vi "Control - X-tau.vi"(8 "Control Inputs":T1 {"CA50 Control Output [CAD]" format="%.2f"; "Exhaust Manifold Temp [C]" format="%#_6f"; "UEGO2Lambda" format="%.2f"; "Intake Manifold Temp (MAT) [C]" format="%#_6f"; "UEGO1Lambda" format="%.2f"}, 11 "Fuel Mass [mg/cyc]":sgl) -> (3 "Fuel Mass [mg/cyc]":sgl)   [LabVIEW 2015, in "ECS-RT.lvlib"]
uses:
  ECS-RT.lvlib
  Typedefs/Control Inputs/Control Inputs.ctl
  Typedefs/EPT/Engine Status.ctl
  Typedefs/MISC/Load Control Mode.ctl
  ECS-Shared.lvlib
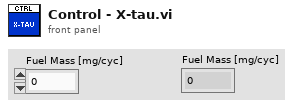
[diagram p1: front panel]
types:
  T1 = typedef "ECS-Shared.lvlib/Control Inputs.ctl" = cluster{"Engine Speed [RPM]":sgl, "Engine Status":T2, "Load Control \nMode":T3, "dt(s)":sgl, "Number of Cylinders":u8, "Engine Displacement [cc]":sgl, "StoichAFR":sgl, "Q.LHV Fuel [kJ/kg]":sgl, "BattV PSU [V]":sgl, "12V PSU [V]":sgl, "5V PSU [V]":sgl, "Pedal Position [%]":sgl, "Oil Pressure [kPa]":sgl, "Oil Temp [C]":sgl, "Oil Level [%]":sgl, "Engine Coolant Temp (ECT) [C]":sgl, "Engine Coolant Pressure [kPa]":sgl, "Rail Pressure [bar]":sgl, "Fuel Pressure [kPa]":sgl, "Fuel Temp [C]":sgl, "Vacuum Pressure [kPa]":sgl, "Throttle Position [%]":sgl, "Cam1 Advance [CAD]":sgl, "Cam2 Advance [CAD]":sgl, "CA50 Control Output [CAD]":sgl[], "CA50 Control Output Valid":bool[], "Intake Air Temp (IAT) [C]":sgl, "Barometric Air Pressure [kPa]":sgl, "Intake Air Rel. Humidity [%]":sgl, "Mass Air Flow (MAF) [kg/hr]":sgl, "Turbo Inlet Air Pressure [kPa]":sgl, "Turbo Inlet Air Temp [C]":sgl, "Turbo Outlet Air Pressure [kPa]":sgl, "Turbo Outlet Air Temp [C]":sgl, "CAC Outlet Pressure [kPa]":sgl, "CAC Outlet Temp [C]":sgl, "Intake Manifold Pressure (MAP) [kPa]":sgl, "Intake Manifold Temp (MAT) [C]":sgl, "Exhaust Manifold Pressure [kPa]":sgl, "Exhaust Manifold Temp [C]":sgl, "HighP EGR Cooler Outlet Pressure [kPa]":sgl, "HighP EGR Cooler Outlet Temp [C]":sgl, "HighP EGR Differential Pressure [kPa]":sgl, "HighP EGR Valve Position [%]":sgl, "Turbo Outlet Exhaust Pressure [kPa]":sgl, "Turbo Outlet Exhaust Temp [C]":sgl, "VGT Position 1 [%]":sgl, "VGT Position 2 [%]":sgl, "Turbo Speed 1 [RPM]":sgl, "Turbo Speed 2 [RPM]":sgl, "LowP EGR Differential Pressure [kPa]":sgl, "LowP EGR Valve Position [%]":sgl, "UEGO1Lambda":sgl, "UEGO1_Hot":bool, "UEGO2Lambda":sgl, "UEGO2_Hot":bool}
  T2 = typedef "ECS-Shared.lvlib/Engine Status.ctl" = enum16{"STALLED", "CRANKING", "RUNNING", "ACCEL", "DECEL", "SAFE", "OFF"}
  T3 = typedef "ECS-Shared.lvlib/Load Control Mode.ctl" = enum16{"No Governor", "Low-Idle Governor", "High-Idle Governor"}
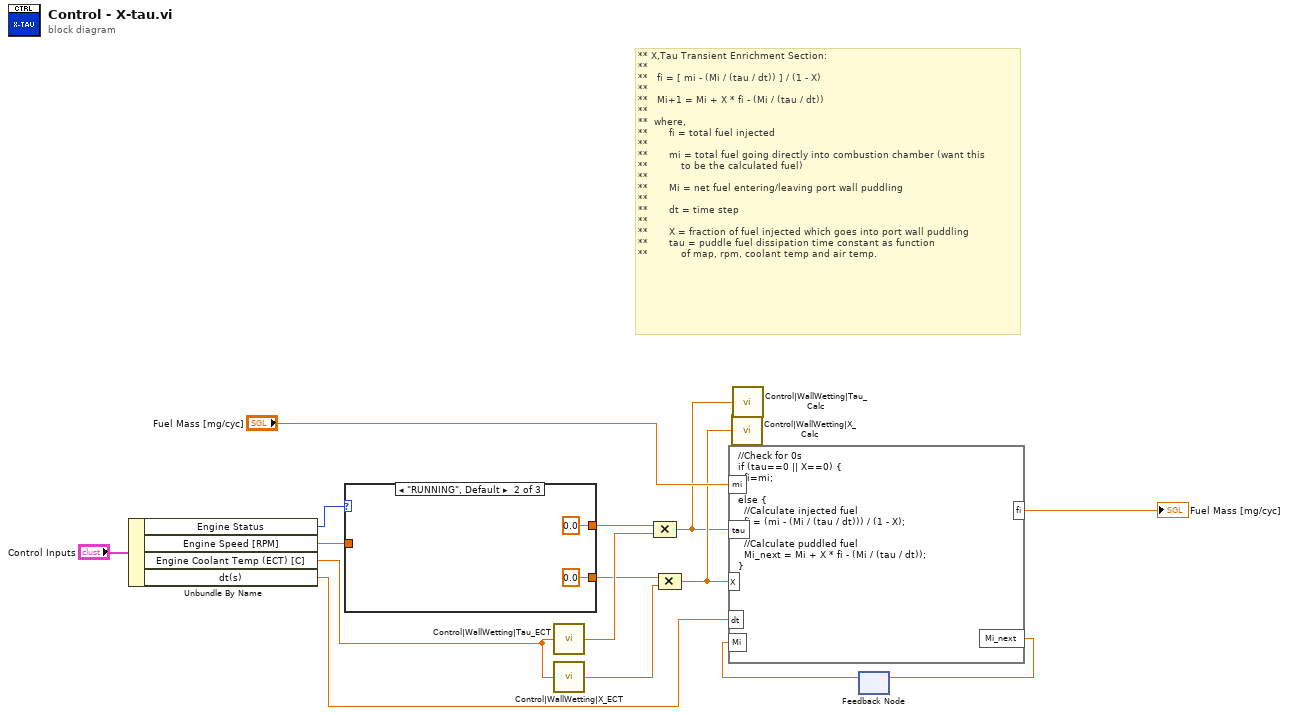
[diagram p0: block diagram]
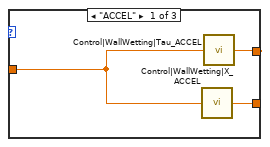
[diagram p2: hidden frame]
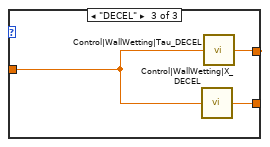
[diagram p3: hidden frame]
diagram:
  # "** X,Tau Transient Enrichment Section:\n**   \n**   fi = [ mi - (Mi / (tau / dt)) ] / (1 - X)\n**\n**   Mi+1 = Mi + X * fi - (Mi / (tau / dt))\n**\n**  where,\n**       fi = total fuel injected\n**\n**       mi = total fuel going directly into combustion chamber (want this \n**           to be the calculated fuel)\n**       \n**       Mi = net fuel entering/leaving port wall puddling\n**       \n**       dt = time step\n**\n**       X = fraction of fuel injected which goes into port wall puddling\n**       tau = puddle fuel dissipation time constant as function \n**           of map, rpm, coolant temp and air temp."
  n1 = Unbundle By Name("Control Inputs") -> ("Engine Status"=w1:T2, "Engine Speed [RPM]"=w4:sgl, "Engine Coolant Temp (ECT) [C]"=w3:sgl, "dt(s)"=w2:sgl)
  n2 = case shown="\"RUNNING\", Default" w1 {
    tunnel: [w18 sgl 0.0 ("Y") w23] -> w6
    tunnel: [w17 sgl 0.0 ("Y") w22] -> w5
    tunnel: w4 -> [w16 _ w21]
    frame "ACCEL" {
      n3 = call "Control|WallWetting|X_ACCEL"("X Index"=w16) -> ("Y"=w17:sgl)
      n4 = call "Control|WallWetting|Tau_ACCEL"("X Index"=w16) -> ("Y"=w18:sgl)
    }
    frame "RUNNING", Default {
    }
    frame "DECEL" {
      n5 = call "Control|WallWetting|X_DECEL"("X Index"=w21) -> ("Y"=w22:sgl)
      n6 = call "Control|WallWetting|Tau_DECEL"("X Index"=w21) -> ("Y"=w23:sgl)
    }
  }
  n7 = call "Control|WallWetting|Tau_ECT"("X Index"=w3) -> ("Y"=w7:sgl)
  n8 = call "Control|WallWetting|X_ECT"("X Index"=w3) -> ("Y"=w10:sgl)
  n9 = Compound Arithmetic op=MULTIPLY(w6, w7) -> (w8:sgl)
  n10 = Compound Arithmetic op=MULTIPLY(w5, w10) -> (w9:sgl)
  n11 = call "Control|WallWetting|X_Calc"("Value"=w9) -> ()
  n12 = call "Control|WallWetting|Tau_Calc"("Value"=w8) -> ()
  n13 = feedback #1() -> (w12:dbl)  [unwired: 1 in]
  n14 = formula code="//Check for 0s\nif (tau==0 || X==0) {\n  fi=mi;\n}\nelse {\n  //Calculate injected fuel\n  fi = (mi - (Mi / (tau / dt))) / (1 - X);\n\n  //Calculate puddled fuel\n  Mi_next = Mi + X * fi - (Mi / (tau / dt));\n}"("tau"=w8, "X"=w9, "mi"="Fuel Mass [mg/cyc]", "dt"=w2, "Mi"=w12) -> ("Mi_next"=w13:dbl, "fi"=→"Fuel Mass [mg/cyc]":dbl)
  n15 = feedback-in #1(w13) -> ()
